vi "VISJS Viewer.vi"(4 "Extra Scripts":string, 5 "FileDependency out":map{path, T1}(c390), 6 "Options":string, 7 "OpenWebBrowser(False)":bool, 8 "error in":errorcluster, 9 "Embedd VISJS Librarya in HTMl File(False)":bool, 10 "HTMLFilePath":path, 11 "LibraryDependency":map{path, T3}(c390)) -> (0 "error out":errorcluster, 3 "HTMLFileContent":string)   [LabVIEW 2020, in "VISJS Viewer.lvlib"] (continued)
t.promise}});var kE=mE,xE=ll;!function(g){var t=db.default,A=wn,e=cd,C=qm,I=ib,i=hb,o=Ld,n=gb,r=kE,s=xE,a=rh;function d(){g.exports=d=function(){return l},g.exports.__esModule=!0,g.exports.default=g.exports;var h,l={},c=Object.prototype,u=c.hasOwnProperty,p=A||function(g,t,A){g[t]=A.value},f=\"function\"==typeof e?e:{},v=f.iterator||\"@@iterator\",y=f.asyncIterator||\"@@asyncIterator\",m=f.toStringTag||\"@@toStringTag\";function b(g,t,e){return A(g,t,{value:e,enumerable:!0,configurable:!0,writable:!0}),g[t]}try{b({},\"\")}catch(h){b=function(g,t,A){return g[t]=A}}function w(g,t,A,e){var I=t&&t.prototype instanceof N?t:N,i=C(I.prototype),o=new V(e||[]);return p(i,\"_invoke\",{value:F(g,A,o)}),i}function k(g,t,A){try{return{type:\"normal\",arg:g.call(t,A)}}catch(g){return{type:\"throw\",arg:g}}}l.wrap=w;var x=\"suspendedStart\",E=\"suspendedYield\",O=\"executing\",T=\"completed\",D={};function N(){}function R(){}function P(){}var M={};b(M,v,(function(){return this}));var B=I&&I(I(Y([])));B&&B!==c&&u.call(B,v)&&(M=B);var z=P.prototype=N.prototype=C(M);function S(g){var t;i(t=[\"next\",\"throw\",\"return\"]).call(t,(function(t){b(g,t,(function(g){return this._invoke(t,g)}))}))}function Z(g,A){function e(C,I,i,o){var n=k(g[C],g,I);if(\"throw\"!==n.type){var r=n.arg,s=r.value;return s&&\"object\"==t(s)&&u.call(s,\"__await\")?A.resolve(s.__await).then((function(g){e(\"next\",g,i,o)}),(function(g){e(\"throw\",g,i,o)})):A.resolve(s).then((function(g){r.value=g,i(r)}),(function(g){return e(\"throw\",g,i,o)}))}o(n.arg)}var C;p(this,\"_invoke\",{value:function(g,t){function I(){return new A((function(A,C){e(g,t,A,C)}))}return C=C?C.then(I,I):I()}})}function F(g,t,A){var e=x;return function(C,I){if(e===O)throw new Error(\"Generator is already running\");if(e===T){if(\"throw\"===C)throw I;return{value:h,done:!0}}for(A.method=C,A.arg=I;;){var i=A.delegate;if(i){var o=G(i,A);if(o){if(o===D)continue;return o}}if(\"next\"===A.method)A.sent=A._sent=A.arg;else if(\"throw\"===A.method){if(e===x)throw e=T,A.arg;A.dispatchException(A.arg)}else\"return\"===A.method&&A.abrupt(\"return\",A.arg);e=O;var n=k(g,t,A);if(\"normal\"===n.type){if(e=A.done?T:E,n.arg===D)continue;return{value:n.arg,done:A.done}}\"throw\"===n.type&&(e=T,A.method=\"throw\",A.arg=n.arg)}}}function G(g,t){var A=t.method,e=g.iterator[A];if(e===h)return t.delegate=null,\"throw\"===A&&g.iterator.return&&(t.method=\"return\",t.arg=h,G(g,t),\"throw\"===t.method)||\"return\"!==A&&(t.method=\"throw\",t.arg=new TypeError(\"The iterator does not provide a '\"+A+\"' method\")),D;var C=k(e,g.iterator,t.arg);if(\"throw\"===C.type)return t.method=\"throw\",t.arg=C.arg,t.delegate=null,D;var I=C.arg;return I?I.done?(t[g.resultName]=I.value,t.next=g.nextLoc,\"return\"!==t.method&&(t.method=\"next\",t.arg=h),t.delegate=null,D):I:(t.method=\"throw\",t.arg=new TypeError(\"iterator result is not an object\"),t.delegate=null,D)}function j(g){var t,A={tryLoc:g[0]};1 in g&&(A.catchLoc=g[1]),2 in g&&(A.finallyLoc=g[2],A.afterLoc=g[3]),o(t=this.tryEntries).call(t,A)}function L(g){var t=g.completion||{};t.type=\"normal\",delete t.arg,g.completion=t}function V(g){this.tryEntries=[{tryLoc:\"root\"}],i(g).call(g,j,this),this.reset(!0)}function Y(g){if(g||\"\"===g){var A=g[v];if(A)return A.call(g);if(\"function\"==typeof g.next)return g;if(!isNaN(g.length)){var e=-1,C=function t(){for(;++e<g.length;)if(u.call(g,e))return t.value=g[e],t.done=!1,t;return t.value=h,t.done=!0,t};return C.next=C}}throw new TypeError(t(g)+\" is not iterable\")}return R.prototype=P,p(z,\"constructor\",{value:P,configurable:!0}),p(P,\"constructor\",{value:R,configurable:!0}),R.displayName=b(P,m,\"GeneratorFunction\"),l.isGeneratorFunction=function(g){var t=\"function\"==typeof g&&g.constructor;return!!t&&(t===R||\"GeneratorFunction\"===(t.displayName||t.name))},l.mark=function(g){return n?n(g,P):(g.__proto__=P,b(g,m,\"GeneratorFunction\")),g.prototype=C(z),g},l.awrap=function(g){return{__await:g}},S(Z.prototype),b(Z.prototype,y,(function(){return this})),l.AsyncIterator=Z,l.async=function(g,t,A,e,C){void 0===C&&(C=r);var I=new Z(w(g,t,A,e),C);return l.isGeneratorFunction(t)?I:I.next().then((function(g){return g.done?g.value:I.next()}))},S(z),b(z,m,\"Generator\"),b(z,v,(function(){return this})),b(z,\"toString\",(function(){return\"[object Generator]\"})),l.keys=function(g){var t=Object(g),A=[];for(var e in t)o(A).call(A,e);return s(A).call(A),function g(){for(;A.length;){var e=A.pop();if(e in t)return g.value=e,g.done=!1,g}return g.done=!0,g}},l.values=Y,V.prototype={constructor:V,reset:function(g){var t;if(this.prev=0,this.next=0,this.sent=this._sent=h,this.done=!1,this.delegate=null,this.method=\"next\",this.arg=h,i(t=this.tryEntries).call(t,L),!g)for(var A in this)\"t\"===A.charAt(0)&&u.call(this,A)&&!isNaN(+a(A).call(A,1))&&(this[A]=h)},stop:function(){this.done=!0;var g=this.tryEntries[0].completion;if(\"throw\"===g.type)throw g.arg;return this.rval},dispatchException:function(g){if(this.done)throw g;var t=this;function A(A,e){return I.type=\"throw\",I.arg=g,t.next=A,e&&(t.method=\"next\",t.arg=h),!!e}for(var e=this.tryEntries.length-1;e>=0;--e){var C=this.tryEntries[e],I=C.completion;if(\"root\"===C.tryLoc)return A(\"end\");if(C.tryLoc<=this.prev){var i=u.call(C,\"catchLoc\"),o=u.call(C,\"finallyLoc\");if(i&&o){if(this.prev<C.catchLoc)return A(C.catchLoc,!0);if(this.prev<C.finallyLoc)return A(C.finallyLoc)}else if(i){if(this.prev<C.catchLoc)return A(C.catchLoc,!0)}else{if(!o)throw new Error(\"try statement without catch or finally\");if(this.prev<C.finallyLoc)return A(C.finallyLoc)}}}},abrupt:function(g,t){for(var A=this.tryEntries.length-1;A>=0;--A){var e=this.tryEntries[A];if(e.tryLoc<=this.prev&&u.call(e,\"finallyLoc\")&&this.prev<e.finallyLoc){var C=e;break}}C&&(\"break\"===g||\"continue\"===g)&&C.tryLoc<=t&&t<=C.finallyLoc&&(C=null);var I=C?C.completion:{};return I.type=g,I.arg=t,C?(this.method=\"next\",this.next=C.finallyLoc,D):this.complete(I)},complete:function(g,t){if(\"throw\"===g.type)throw g.arg;return\"break\"===g.type||\"continue\"===g.type?this.next=g.arg:\"return\"===g.type?(this.rval=this.arg=g.arg,this.method=\"return\",this.next=\"end\"):\"normal\"===g.type&&t&&(this.next=t),D},finish:function(g){for(var t=this.tryEntries.length-1;t>=0;--t){var A=this.tryEntries[t];if(A.finallyLoc===g)return this.complete(A.completion,A.afterLoc),L(A),D}},catch:function(g){for(var t=this.tryEntries.length-1;t>=0;--t){var A=this.tryEntries[t];if(A.tryLoc===g){var e=A.completion;if(\"throw\"===e.type){var C=e.arg;L(A)}return C}}throw new Error(\"illegal catch attempt\")},delegateYield:function(g,t,A){return this.delegate={iterator:Y(g),resultName:t,nextLoc:A},\"next\"===this.method&&(this.arg=h),D}},l}g.exports=d,g.exports.__esModule=!0,g.exports.default=g.exports}(sb);var EE=(0,sb.exports)(),OE=EE;try{regeneratorRuntime=EE}catch(g){\"object\"==typeof globalThis?globalThis.regeneratorRuntime=EE:Function(\"r\",\"regeneratorRuntime = r\")(EE)}var TE=A(OE),DE=Rg,NE=Hg,RE=W,PE=jA,ME=TypeError,BE=function(g){return function(t,A,e,C){DE(A);var I=NE(t),i=RE(I),o=PE(I),n=g?o-1:0,r=g?-1:1;if(e<2)for(;;){if(n in i){C=i[n],n+=r;break}if(n+=r,g?n<0:o<=n)throw new ME(\"Reduce of empty array with no initial value\")}for(;g?n>=0:o>n;n+=r)n in i&&(C=A(C,i[n],n,I));return C}},zE={left:BE(!1),right:BE(!0)}.left;TA({target:\"Array\",proto:!0,forced:!$b&&cg>79&&cg<83||!_h(\"reduce\")},{reduce:function(g){var t=arguments.length;return zE(this,g,t,t>1?arguments[1]:void 0)}});var SE=Me(\"Array\").reduce,ZE=og,FE=SE,GE=Array.prototype,jE=function(g){var t=g.reduce;return g===GE||ZE(GE,g)&&t===GE.reduce?FE:t},LE=A(jE),VE=En,YE=jA,WE=Tn,QE=Xt,UE=function(g,t,A,e,C,I,i,o){for(var n,r,s=C,a=0,d=!!i&&QE(i,o);a<e;)a in A&&(n=d?d(A[a],a,t):A[a],I>0&&VE(n)?(r=YE(n),s=UE(g,t,n,r,s,I-1)-1):(WE(s+1),g[s]=n),s++),a++;return s},_E=UE,KE=Rg,HE=Hg,XE=jA,JE=zn;TA({target:\"Array\",proto:!0},{flatMap:function(g){var t,A=HE(this),e=XE(A);return KE(g),(t=JE(A,0)).length=_E(t,A,A,e,0,1,g,arguments.length>1?arguments[1]:void 0),t}});var qE=Me(\"Array\").flatMap,$E=og,gO=qE,tO=Array.prototype,AO=function(g){var t=g.flatMap;return g===tO||$E(tO,g)&&t===tO.flatMap?gO:t},eO=A(AO);cm(\"Set\",(function(g){return function(){return g(this,arguments.length?arguments[0]:void 0)}}),Zm);var CO=A(tg.Set),IO=A(pd),iO=A(Oo),oO=rr,nO=Math.floor,rO=function(g,t){var A=g.length,e=nO(A/2);return A<8?sO(g,t):aO(g,rO(oO(g,0,e),t),rO(oO(g,e),t),t)},sO=function(g,t){for(var A,e,C=g.length,I=1;I<C;){for(e=I,A=g[I];e&&t(g[e-1],A)>0;)g[e]=g[--e];e!==I++&&(g[e]=A)}return g},aO=function(g,t,A,e){for(var C=t.length,I=A.length,i=0,o=0;i<C||o<I;)g[i+o]=i<C&&o<I?e(t[i],A[o])<=0?t[i++]:A[o++]:i<C?t[i++]:A[o++];return g},dO=rO,hO=ng.match(/firefox\\/(\\d+)/i),lO=!!hO&&+hO[1],cO=/MSIE|Trident/.test(ng),uO=ng.match(/AppleWebKit\\/(\\d+)\\./),pO=!!uO&&+uO[1],fO=TA,vO=u,yO=Rg,mO=Hg,bO=jA,wO=fl,kO=sC,xO=I,EO=dO,OO=_h,TO=lO,DO=cO,NO=cg,RO=pO,PO=[],MO=vO(PO.sort),BO=vO(PO.push),zO=xO((function(){PO.sort(void 0)})),SO=xO((function(){PO.sort(null)})),ZO=OO(\"sort\"),FO=!xO((function(){if(NO)return NO<70;if(!(TO&&TO>3)){if(DO)return!0;if(RO)return RO<603;var g,t,A,e,C=\"\";for(g=65;g<76;g++){switch(t=String.fromCharCode(g),g){case 66:case 69:case 70:case 72:A=3;break;case 68:case 71:A=4;break;default:A=2}for(e=0;e<47;e++)PO.push({k:t+e,v:A})}for(PO.sort((function(g,t){return t.v-g.v})),e=0;e<PO.length;e++)t=PO[e].k.charAt(0),C.charAt(C.length-1)!==t&&(C+=t);return\"DGBEFHACIJK\"!==C}}));fO({target:\"Array\",proto:!0,forced:zO||!SO||!ZO||!FO},{sort:function(g){void 0!==g&&yO(g);var t=mO(this);if(FO)return void 0===g?MO(t):MO(t,g);var A,e,C=[],I=bO(t);for(e=0;e<I;e++)e in t&&BO(C,t[e]);for(EO(C,function(g){return function(t,A){return void 0===A?-1:void 0===t?1:void 0!==g?+g(t,A)||0:kO(t)>kO(A)?1:-1}}(g)),A=bO(C),e=0;e<A;)t[e]=C[e++];for(;e<I;)wO(t,e++);return t}});var GO=Me(\"Array\").sort,jO=og,LO=GO,VO=Array.prototype,YO=function(g){var t=g.sort;return g===VO||jO(VO,g)&&t===VO.sort?LO:t},WO=A(YO),QO=Me(\"Array\").keys,UO=oC,_O=qg,KO=og,HO=QO,XO=Array.prototype,JO={DOMTokenList:!0,NodeList:!0},qO=function(g){var t=g.keys;return g===XO||KO(XO,g)&&t===XO.keys||_O(JO,UO(g))?HO:t},$O=A(qO),gT=Me(\"Array\").values,tT=oC,AT=qg,eT=og,CT=gT,IT=Array.prototype,iT={DOMTokenList:!0,NodeList:!0},oT=function(g){var t=g.values;return g===IT||eT(IT,g)&&t===IT.values||AT(iT,tT(g))?CT:t},nT=A(oT),rT=Me(\"Array\").entries,sT=oC,aT=qg,dT=og,hT=rT,lT=Array.prototype,cT={DOMTokenList:!0,NodeList:!0},uT=function(g){var t=g.entries;return g===lT||dT(lT,g)&&t===lT.entries||aT(cT,sT(g))?hT:t},pT=A(uT),fT=A(bn),vT=TA,yT=a,mT=Ne,bT=ew,wT=AA,kT=gg,xT=pI,ET=I,OT=ig(\"Reflect\",\"construct\"),TT=Object.prototype,DT=[].push,NT=ET((function(){function g(){}return!(OT((function(){}),[],g)instanceof g)})),RT=!ET((function(){OT((function(){}))})),PT=NT||RT;vT({target:\"Reflect\",stat:!0,forced:PT,sham:PT},{construct:function(g,t){bT(g),wT(t);var A=arguments.length<3?g:bT(arguments[2]);if(RT&&!NT)return OT(g,t,A);if(g===A){switch(t.length){case 0:return new g;case 1:return new g(t[0]);case 2:return new g(t[0],t[1]);case 3:return new g(t[0],t[1],t[2]);case 4:return new g(t[0],t[1],t[2],t[3])}var e=[null];return yT(DT,e,t),new(yT(mT,g,e))}var C=A.prototype,I=xT(kT(C)?C:TT),i=yT(g,I,t);return kT(i)?i:I}});var MT=A(tg.Reflect.construct),BT=A(tg.Object.getOwnPropertySymbols),zT={exports:{}},ST=TA,ZT=I,FT=J,GT=T.f,jT=D;ST({target:\"Object\",stat:!0,forced:!jT||ZT((function(){GT(1)})),sham:!jT},{getOwnPropertyDescriptor:function(g,t){return GT(FT(g),t)}});var LT=tg.Object,VT=zT.exports=function(g,t){return LT.getOwnPropertyDescriptor(g,t)};LT.getOwnPropertyDescriptor.sham&&(VT.sham=!0);var YT=zT.exports,WT=A(YT),QT=Dh,UT=J,_T=T,KT=lo;TA({target:\"Object\",stat:!0,sham:!D},{getOwnPropertyDescriptors:function(g){for(var t,A,e=UT(g),C=_T.f,I=QT(e),i={},o=0;I.length>o;)void 0!==(A=C(e,t=I[o++]))&&KT(i,t,A);return i}});var HT=A(tg.Object.getOwnPropertyDescriptors),XT={exports:{}},JT=TA,qT=D,$T=UC.f;JT({target:\"Object\",stat:!0,forced:Object.defineProperties!==$T,sham:!qT},{defineProperties:$T});var gD=tg.Object,tD=XT.exports=function(g,t){return gD.defineProperties(g,t)};gD.defineProperties.sham&&(tD.sham=!0);var AD=A(XT.exports);let eD;const CD=new Uint8Array(16);function ID(){if(!eD&&(eD=\"undefined\"!=typeof crypto&&crypto.getRandomValues&&crypto.getRandomValues.bind(crypto),!eD))throw new Error(\"crypto.getRandomValues() not supported. See https://github.com/uuidjs/uuid#getrandomvalues-not-supported\");return eD(CD)}const iD=[];for(let g=0;g<256;++g)iD.push((g+256).toString(16).slice(1));var oD,nD={randomUUID:\"undefined\"!=typeof crypto&&crypto.randomUUID&&crypto.randomUUID.bind(crypto)};function rD(g,t,A){if(nD.randomUUID&&!t&&!g)return nD.randomUUID();const e=(g=g||{}).random||(g.rng||ID)();if(e[6]=15&e[6]|64,e[8]=63&e[8]|128,t){A=A||0;for(let g=0;g<16;++g)t[A+g]=e[g];return t}return function(g,t=0){return iD[g[t+0]]+iD[g[t+1]]+iD[g[t+2]]+iD[g[t+3]]+\"-\"+iD[g[t+4]]+iD[g[t+5]]+\"-\"+iD[g[t+6]]+iD[g[t+7]]+\"-\"+iD[g[t+8]]+iD[g[t+9]]+\"-\"+iD[g[t+10]]+iD[g[t+11]]+iD[g[t+12]]+iD[g[t+13]]+iD[g[t+14]]+iD[g[t+15]]}(e)}function sD(g,t){var A=Lh(g);if(BT){var e=BT(g);t&&(e=pc(e).call(e,(function(t){return WT(g,t).enumerable}))),A.push.apply(A,e)}return A}function aD(g){for(var t=1;t<arguments.length;t++){var A,e,C=null!=arguments[t]?arguments[t]:{};t%2?Cl(A=sD(Object(C),!0)).call(A,(function(t){rb(g,t,C[t])})):HT?AD(g,HT(C)):Cl(e=sD(Object(C))).call(e,(function(t){fT(g,t,WT(C,t))}))}return g}function dD(g){var t=function(){if(\"undefined\"==typeof Reflect||!MT)return!1;if(MT.sham)return!1;if(\"function\"==typeof Proxy)return!0;try{return Boolean.prototype.valueOf.call(MT(Boolean,[],(function(){}))),!0}catch(g){return!1}}();return function(){var A,e=nb(g);if(t){var C=nb(this).constructor;A=MT(e,arguments,C)}else A=e.apply(this,arguments);return Ib(this,A)}}function hD(g,t){var A=void 0!==uh&&ln(g)||g[\"@@iterator\"];if(!A){if(Rh(g)||(A=function(g,t){var A;if(!g)return;if(\"string\"==typeof g)return lD(g,t);var e=wh(A=Object.prototype.toString.call(g)).call(A,8,-1);\"Object\"===e&&g.constructor&&(e=g.constructor.name);if(\"Map\"===e||\"Set\"===e)return Uo(g);if(\"Arguments\"===e||/^(?:Ui|I)nt(?:8|16|32)(?:Clamped)?Array$/.test(e))return lD(g,t)}(g))||t&&g&&\"number\"==typeof g.length){A&&(g=A);var e=0,C=function(){};return{s:C,n:function(){return e>=g.length?{done:!0}:{done:!1,value:g[e++]}},e:function(g){throw g},f:C}}throw new TypeError(\"Invalid attempt to iterate non-iterable instance.\\nIn order to be iterable, non-array objects must have a [Symbol.iterator]() method.\")}var I,i=!0,o=!1;return{s:function(){A=A.call(g)},n:function(){var g=A.next();return i=g.done,g},e:function(g){o=!0,I=g},f:function(){try{i||null==A.return||A.return()}finally{if(o)throw I}}}}function lD(g,t){(null==t||t>g.length)&&(t=g.length);for(var A=0,e=new Array(t);A<t;A++)e[A]=g[A];return e}var cD=function(){function g(t,A,e){var C,I,i;cn(this,g),rb(this,\"_source\",void 0),rb(this,\"_transformers\",void 0),rb(this,\"_target\",void 0),rb(this,\"_listeners\",{add:je(C=this._add).call(C,this),remove:je(I=this._remove).call(I,this),update:je(i=this._update).call(i,this)}),this._source=t,this._transformers=A,this._target=e}return kd(g,[{key:\"all\",value:function(){return this._target.update(this._transformItems(this._source.get())),this}},{key:\"start\",value:function(){return this._source.on(\"add\",this._listeners.add),this._source.on(\"remove\",this._listeners.remove),this._source.on(\"update\",this._listeners.update),this}},{key:\"stop\",value:function(){return this._source.off(\"add\",this._listeners.add),this._source.off(\"remove\",this._listeners.remove),this._source.off(\"update\",this._listeners.update),this}},{key:\"_transformItems\",value:function(g){var t;return LE(t=this._transformers).call(t,(function(g,t){return t(g)}),g)}},{key:\"_add\",value:function(g,t){null!=t&&this._target.add(this._transformItems(this._source.get(t.items)))}},{key:\"_update\",value:function(g,t){null!=t&&this._target.update(this._transformItems(this._source.get(t.items)))}},{key:\"_remove\",value:function(g,t){null!=t&&this._target.remove(this._transformItems(t.oldData))}}]),g}(),uD=function(){function g(t){cn(this,g),rb(this,\"_source\",void 0),rb(this,\"_transformers\",[]),this._source=t}return kd(g,[{key:\"filter\",value:function(g){return this._transformers.push((function(t){return pc(t).call(t,g)})),this}},{key:\"map\",value:function(g){return this._transformers.push((function(t){return Fh(t).call(t,g)})),this}},{key:\"flatMap\",value:function(g){return this._transformers.push((function(t){return eO(t).call(t,g)})),this}},{key:\"to\",value:function(g){return new cD(this._source,this._transformers,g)}}]),g}();function pD(g){return\"string\"==typeof g||\"number\"==typeof g}var fD=function(){function g(t){cn(this,g),rb(this,\"delay\",void 0),rb(this,\"max\",void 0),rb(this,\"_queue\",[]),rb(this,\"_timeout\",null),rb(this,\"_extended\",null),this.delay=null,this.max=1/0,this.setOptions(t)}return kd(g,[{key:\"setOptions\",value:function(g){g&&void 0!==g.delay&&(this.delay=g.delay),g&&void 0!==g.max&&(this.max=g.max),this._flushIfNeeded()}},{key:\"destroy\",value:function(){if(this.flush(),this._extended){for(var g=this._extended.object,t=this._extended.methods,A=0;A<t.length;A++){var e=t[A];e.original?g[e.name]=e.original:delete g[e.name]}this._extended=null}}},{key:\"replace\",value:function(g,t){var A=this,e=g[t];if(!e)throw new Error(\"Method \"+t+\" undefined\");g[t]=function(){for(var g=arguments.length,t=new Array(g),C=0;C<g;C++)t[C]=arguments[C];A.queue({args:t,fn:e,context:this})}}},{key:\"queue\",value:function(g){\"function\"==typeof g?this._queue.push({fn:g}):this._queue.push(g),this._flushIfNeeded()}},{key:\"_flushIfNeeded\",value:function(){var g=this;this._queue.length>this.max&&this.flush(),null!=this._timeout&&(clearTimeout(this._timeout),this._timeout=null),this.queue.length>0&&\"number\"==typeof this.delay&&(this._timeout=wu((function(){g.flush()}),this.delay))}},{key:\"flush\",value:function(){var g,t;Cl(g=Zl(t=this._queue).call(t,0)).call(g,(function(g){g.fn.apply(g.context||g.fn,g.args||[])}))}}],[{key:\"extend\",value:function(t,A){var e=new g(A);if(void 0!==t.flush)throw new Error(\"Target object already has a property flush\");t.flush=function(){e.flush()};var C=[{name:\"flush\",original:void 0}];if(A&&A.replace)for(var I=0;I<A.replace.length;I++){var i=A.replace[I];C.push({name:i,original:t[i]}),e.replace(t,i)}return e._extended={object:t,methods:C},e}}]),g}(),vD=function(){function g(){cn(this,g),rb(this,\"_subscribers\",{\"*\":[],add:[],remove:[],update:[]}),rb(this,\"subscribe\",g.prototype.on),rb(this,\"unsubscribe\",g.prototype.off)}return kd(g,[{key:\"_trigger\",value:function(g,t,A){var e,C;if(\"*\"===g)throw new Error(\"Cannot trigger event *\");Cl(e=bh(C=[]).call(C,ch(this._subscribers[g]),ch(this._subscribers[\"*\"]))).call(e,(function(e){e(g,t,null!=A?A:null)}))}},{key:\"on\",value:function(g,t){\"function\"==typeof t&&this._subscribers[g].push(t)}},{key:\"off\",value:function(g,t){var A;this._subscribers[g]=pc(A=this._subscribers[g]).call(A,(function(g){return g!==t}))}}]),g}();oD=IO;var yD=function(){function g(t){cn(this,g),rb(this,\"_pairs\",void 0),this._pairs=t}return kd(g,[{key:oD,value:TE.mark((function g(){var t,A,e,C,I;return TE.wrap((function(g){for(;;)switch(g.prev=g.next){case 0:t=hD(this._pairs),g.prev=1,t.s();case 3:if((A=t.n()).done){g.next=9;break}return e=lh(A.value,2),C=e[0],I=e[1],g.next=7,[C,I];case 7:g.next=3;break;case 9:g.next=14;break;case 11:g.prev=11,g.t0=g.catch(1),t.e(g.t0);case 14:return g.prev=14,t.f(),g.finish(14);case 17:case\"end\":return g.stop()}}),g,this,[[1,11,14,17]])}))},{key:\"entries\",value:TE.mark((function g(){var t,A,e,C,I;return TE.wrap((function(g){for(;;)switch(g.prev=g.next){case 0:t=hD(this._pairs),g.prev=1,t.s();case 3:if((A=t.n()).done){g.next=9;break}return e=lh(A.value,2),C=e[0],I=e[1],g.next=7,[C,I]
